vi "RandomString.vi"() -> (2 "Random String":string)   [LabVIEW 2020, in "VIDiffUtilities.lvlib"]
uses:
  VIDiffUtilities.lvlib
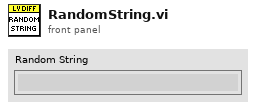
[diagram p1: front panel]
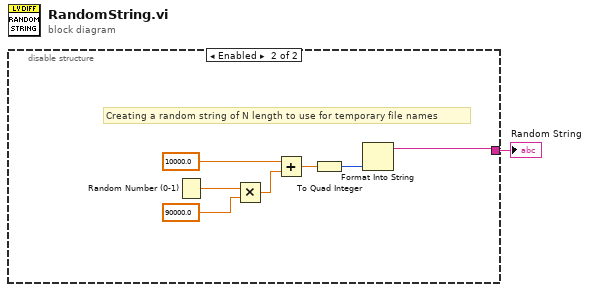
[diagram p0: block diagram]
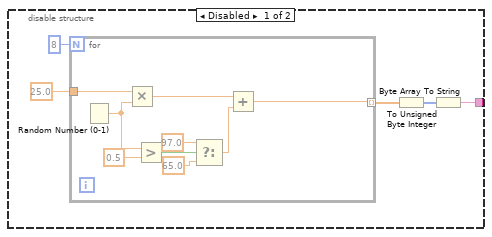
[diagram p2: hidden frame]
diagram:
  n1 = disable-structure shown="Enabled" {
    disable-tunnel: [w2 w16] -> w1
    frame Disabled {
      n2 = for {
        N: 8 -> [_]
        tunnel: 25.0 -> [w14]
        tunnel: [w13] -> w4 mode=indexing
        n3 = Random Number (0-1)() -> (number: 0 to 1=w12:dbl)
        n4 = Multiply(x=w14, y=w12) -> (x*y=w15:dbl)
        n5 = Greater?(x=w12, y=0.5) -> (0:w10:bool)
        n6 = Select(t=97.0, s=w10, f=65.0) -> (s? t:f=w7:dbl)
        n7 = Add(x=w15, y=w7) -> (x+y=w13:dbl)
      }
      n8 = To Unsigned Byte Integer(number=w4) -> (unsigned 8bit integer=w3:u8[])
      n9 = Byte Array To String(unsigned byte array=w3) -> (string=w2:string)
    }
    frame Enabled {
      # "Creating a random string of N length to use for temporary file names"
      n10 = Random Number (0-1)() -> (number: 0 to 1=w22:dbl)
      n11 = Multiply(x=w22, y=90000.0) -> (x*y=w19:dbl)
      n12 = Add(x=10000.0, y=w19) -> (x+y=w18:dbl)
      n13 = To Quad Integer(1:w18) -> (0:w17:i64)
      n14 = Format Into String(w17) -> (resulting string=w16:string)  [unwired: 3 in, 1 out]
    }
  }
  "Random String" <- w1
